vi "test_Set and Get 9474.vi"(8 "error in (no error)":errorcluster, 11 "TestCase in":refnum<class "Scan Engine Scripting API Custom Device Unit Tests.lvclass">) -> (0 "error out":errorcluster, 3 "TestCase out":refnum<class "Scan Engine Scripting API Custom Device Unit Tests.lvclass">)   [LabVIEW 2019, in "Scan Engine Scripting API Custom Device Unit Tests.lvclass"]
uses:
  Scan Engine Scripting API Custom Device Unit Tests.lvclass
  <vilib>/addons/_JKI Toolkits/VI Tester/TestCase.llb/TestCase.lvclass
  Scripting/Scan Engine Scripting.lvlib
  5525f2fe-c77f-4c69-8da2-db807206c7d6.vi
  Scripting/Modules/NI 9474/NI 9474.lvclass
  C:/Users/nitest/Desktop/Git/niveristand-scan-engine-ethercat-custom-device/Custom Device Source/Scripting/Modules/Module/Module.lvclass
  Scripting/Modules/Mode Classes/Counter Driven Output Mode/Drive from Slot.ctl
  Scripting/Modules/Mode Classes/Counter Driven Output Mode/Counter Driven Output Mode.lvclass
  C:/Program Files (x86)/National Instruments/LabVIEW 2019/vi.lib/addons/_JKI Toolkits/VI Tester/TestCase.llb/TestCase.lvclass
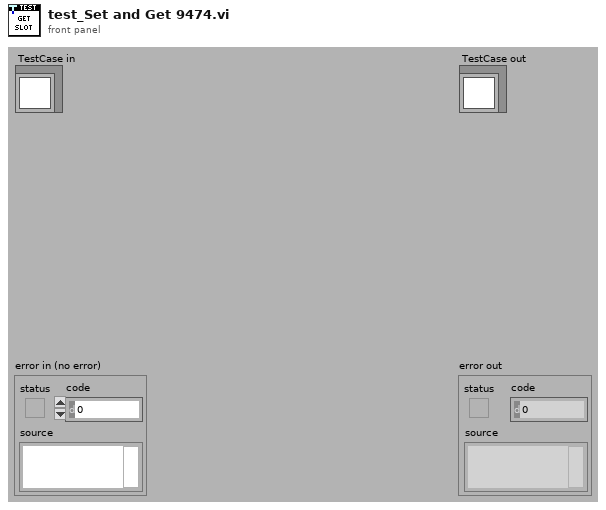
[diagram p1: front panel]
types:
  T1 = typedef "Scan Engine Scripting.lvlib/Counter Driven Output Mode.lvclass/Drive from Slot.ctl" = enum16{"Slot 1", "Slot 2", "Slot 3", "Slot 4", "Slot 5", "Slot 6", "Slot 7", "Slot 8"}
  T2 = typedef "Custom Device API.lvlib/Custom Device Item Ref.ctl" = u64
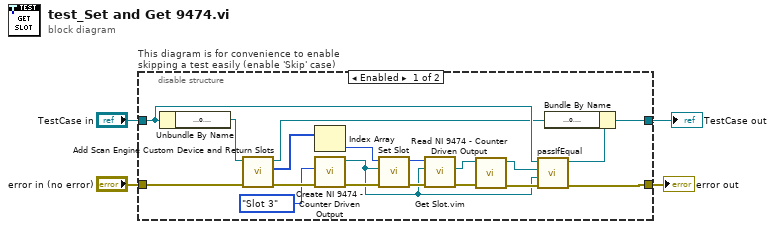
[diagram p0: block diagram]
diagram:
  n1 = disable-structure "This diagram is for convenience to enable skipping a test easily (enable 'Skip' case)" shown="Enabled" {
    disable-tunnel: "TestCase in" -> [w20 w27]
    disable-tunnel: [w22 w25] -> w1
    disable-tunnel: [w18 w26] -> w3
    disable-tunnel: "error in (no error)" -> [w11 w24]
    frame Enabled {
      n2 = Unbundle By Name(w20) -> ("target ref"=w13:refnum<k24>)
      n3 = call "Add Scan Engine Custom Device and Return Slots.vi"("error in"=w11, "target ref in"=w13) -> ("error out"=w10:errorcluster, "slot refs"=w12:T2[], "target ref out"=w9:refnum<k24>)  [unwired: 7 in]
      n4 = Index Array(array=w12) -> (element=w23:T2)  [unwired: 1 in]
      n5 = call "Create NI 9474 - Counter Driven Output.vi"("error in"=w10, "drive from slot"=Drive_from_Slot."Slot 3") -> ("error out"=w19:errorcluster, "NI 9474 out"=w8:refnum<class "NI 9474.lvclass">)  [unwired: 8 in]
      n6 = call "Set Slot.vi"("error in"=w19, "module"=w8, "slot ref in"=w23) -> ("error out"=w21:errorcluster, "slot ref out"=w14:T2)  [unwired: 7 in]
      n7 = call "Get Slot.vim"("error in"=w21, "module type"=w8, "slot ref in"=w14) -> ("error out"=w6:errorcluster, "module"=w7:refnum<class "NI 9474.lvclass">)  [unwired: 5 in, 2 out]
      n8 = call "Read NI 9474 - Counter Driven Output.vi"("error in"=w6, "NI 9474 in"=w7) -> ("error out"=w16:errorcluster, "NI 9474 out"=w17:refnum<class "NI 9474.lvclass">)  [unwired: 6 in, 2 out]
      n9 = call-dynamic "passIfEqual.vi"("error in (no error)"=w16, "y"=w8, "x"=w17, "TestCase in"=w20) -> ("error out"=w18:errorcluster, "TestCase out"=w15:refnum<class "Scan Engine Scripting API Custom Device Unit Tests.lvclass">)  [unwired: 6 in]
      n10 = Bundle By Name(cluster=w15, "target ref"=w9) -> (w22:refnum<class "Scan Engine Scripting API Custom Device Unit Tests.lvclass">)
    }
    frame Disabled {
      # "skip test result while test is under development"
      n11 = call <vilib>:"skip.vi"("error in (no error)"=w24, "TestCase in"=w27) -> ("error out"=w26:errorcluster, "TestCase out"=w25:refnum<class "Scan Engine Scripting API Custom Device Unit Tests.lvclass">)  [unwired: 8 in]
    }
  }
  "error out" <- w3
  "TestCase out" <- w1
